vi "AffichageLUT.vi"(1 "Table de couleurs":u32[](array[numeric])) -> (0 "LUT":picture)   [LabVIEW 2020]
doc: "Nom du VI : AffichageLUT\n\nDescription : \nCe vi dessine une LUT dans une image zoomée en x uniquemen. \nPrincipe : Une première boucle for génère 3 rampes de 0 à 255. . \nDans la deuxième boucle for dessine la \" pixelmap \" en utilisant la table de couleur.\n\nVariables d'entrée : Tableau de couleurs, tableau d'entiers non signés de 32 bits. Ce tableau représente la MUT à dessiner. \n\nVariables de sortie : image, cette image représente la LUT."
panel:
  in  "top left point":cluster{i16, i16}
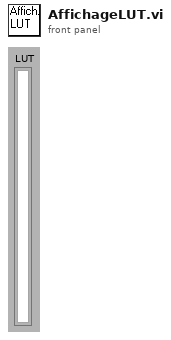
[diagram p1: front panel]
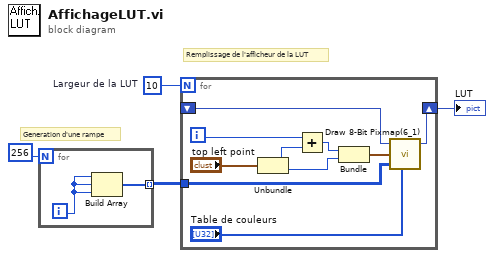
[diagram p0: block diagram]
diagram:
  w3 = 10  # Largeur de la LUT
  # "Remplissage de l'afficheur de la LUT"
  # "Generation d'une rampe"
  n1 = for {
    N: 256 -> [_]
    tunnel: [w6] -> w2 mode=indexing
    i -> [w5]
    n2 = Build Array(w5, w5, w5) -> (w6:i32[])
  }
  n3 = for {
    N: w3 -> [_]
    tunnel: w2 -> [w8]
    shift-right: [w16] -> w1
    shift-left: _ -> [w15]
    i -> [w12]
    n4 = Unbundle("top left point") -> (w13:i16, w10:i16)
    n5 = Add(x=w12, y=w13) -> (x+y=w11:i32)
    n6 = Bundle(w11, w10) -> (w9:cluster{i32, i16})  [unwired: 1 in]
    n7 = call <vilib>:"Draw 8-Bit Pixmap(6_1).vi"("picture"=w15, "top left point(0, 0)"=w9, "data"=w8, "color table"="Table de couleurs") -> ("new picture"=w16:picture)  [unwired: 5 in]
  }
  "LUT" <- w1
